vi "Tree_Get first enabled element from bottom.vi"(8 "error in (no error)":errorcluster, 11 "TreeControl Ref":refnum<vi>) -> (0 "error out":errorcluster, 2 "First Element Tag":string, 3 "Tree Control Ref Out":refnum<vi>)   [LabVIEW 2023]
doc: "Move from bottom of the tree up to find first non-dsiabled item in tree. This will open disabled parent items and traverse their children."
panel:
  in  "Tree":string[](tree)
  # "DEBUG CTRL"
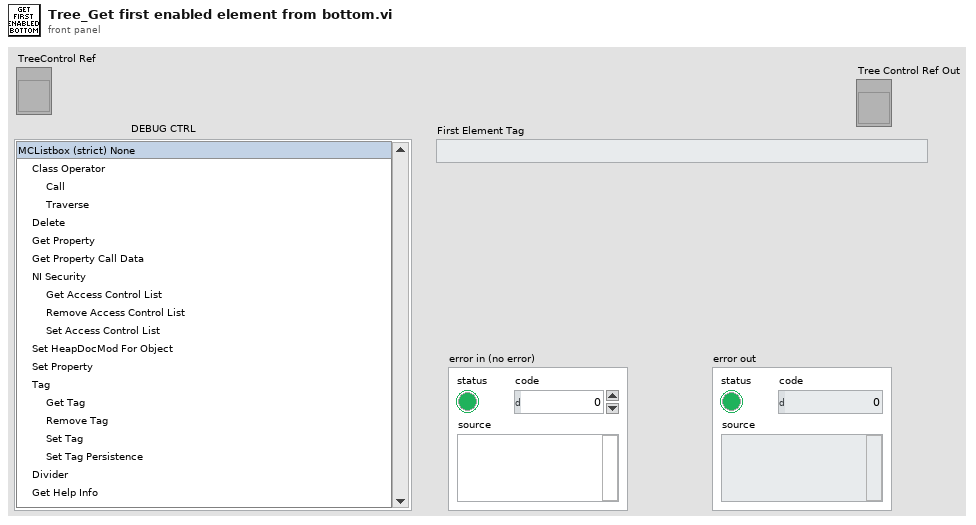
[diagram p1: front panel]
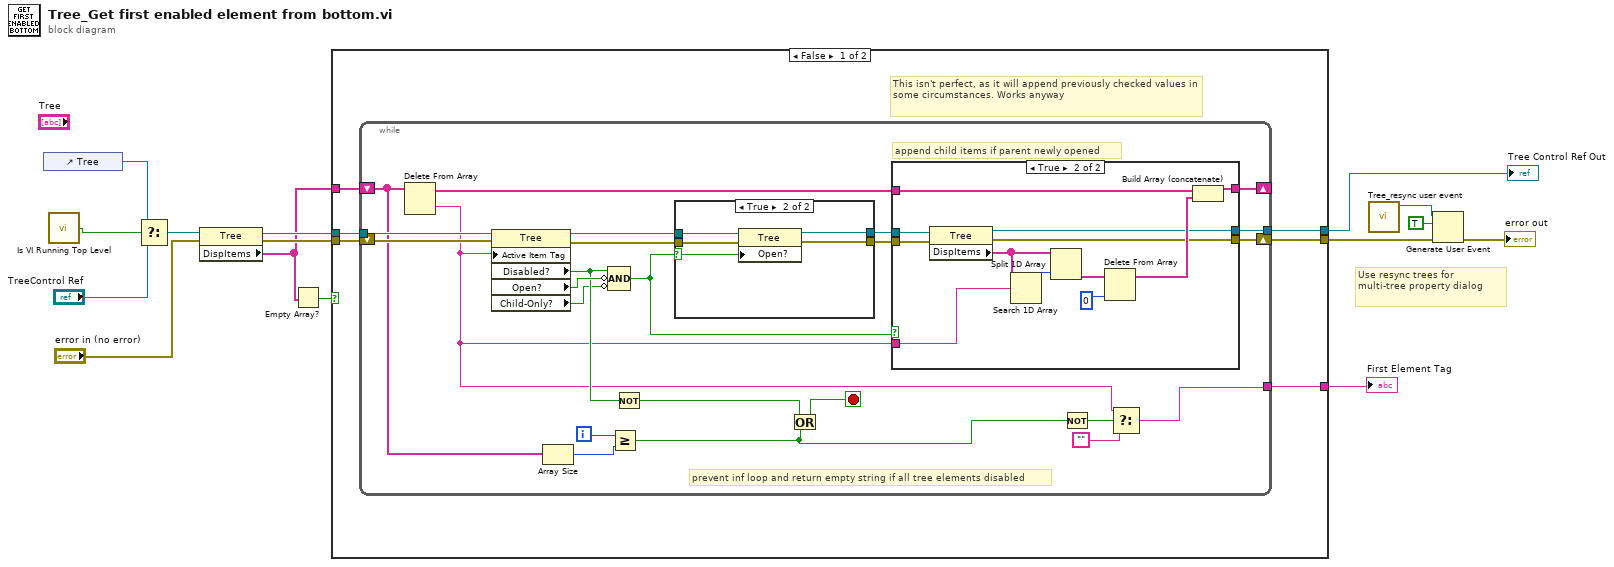
[diagram p0: block diagram]
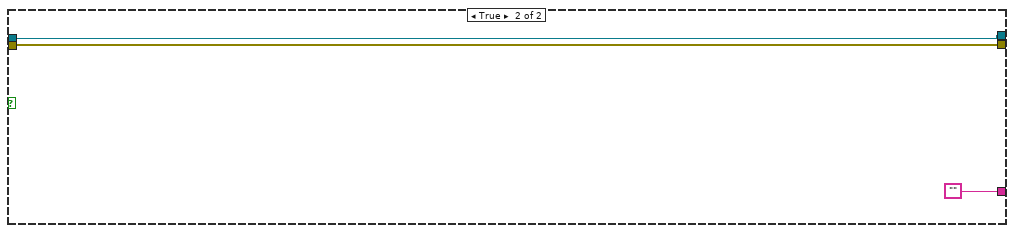
[diagram p4: hidden frame]
diagram:
  # "Use resync trees for multi-tree property dialog"
  n1 = control-ref of="Tree"() -> (w12:refnum<vi>)
  n2 = call "Is VI Running Top Level.vi"() -> ("Top Level?"=w13:bool)  [unwired: 5 in]
  n3 = Select(t=w12, s=w13, f="TreeControl Ref") -> (s? t:f=w10:refnum<vi>)
  n4 = property class="Tree"(reference=w10, error in="error in (no error)") -> (reference out=w15:refnum<vi>, error out=w9:errorcluster, "DispItems"=w2:string[])
  n5 = Empty Array?(array=w2) -> (empty?=w1:bool)
  n6 = case shown="False" w1 {
    tunnel: w15 -> [w21 w70]
    tunnel: w2 -> [w20 _]
    tunnel: [w19 ""] -> w14
    tunnel: w9 -> [w18 w69]
    tunnel: [w17 w70] -> w7
    tunnel: [w16 w69] -> w6
    frame False {
      # "This isn't perfect, as it will append previously checked values in some circumstances. Works anyway"
      n7 = while {
        tunnel: w21 -> [w43]
        tunnel: [w25] -> w19
        shift-right: [w39] -> _
        shift-left: w20 -> [w34]
        shift-right: [w35] -> w16
        shift-left: w18 -> [w38]
        tunnel: [w23] -> w17
        i -> [w33]
        stop <- w30 stop-if-true
        # "append child items if parent newly opened"
        # "prevent inf loop and return empty string if all tree elements disabled"
        n8 = Delete From Array(array=w34) -> (deleted portion=w26:string, array with subset deleted=w40:string[])  [unwired: 2 in]
        n9 = property class="Tree"(reference=w43, error in=w38, "Active Item Tag"=w26) -> (reference out=w45:refnum<vi>, error out=w37:errorcluster, "Disabled?"=w41:bool, "Open?"=w44:bool, "Child-Only?"=w24:bool)
        n10 = Array Size(array=w34) -> (size(s)=w32:i32)
        n11 = Compound Arithmetic op=AND(w41, invert w44, invert w24) -> (w22:bool)
        n12 = Greater Or Equal?(x=w33, y=w32) -> (x >= y?=w29:bool)
        n13 = Not(x=w41) -> (.not. x?=w31:bool)
        n14 = case shown="True" w22 {
          selector: w22 -> [_ w49]
          tunnel: w45 -> [w47 w52]
          tunnel: [w47 w51] -> w42
          tunnel: w37 -> [w46 w50]
          tunnel: [w46 w48] -> w36
          frame False {
          }
          frame True {
            n15 = property class="Tree"(reference=w52, error in=w50, "Open?"=w49) -> (reference out=w51:refnum<vi>, error out=w48:errorcluster)
          }
        }
        n16 = Or(x=w31, y=w29) -> (x .or. y?=w30:bool)
        n17 = case shown="True" w22 {
          tunnel: w42 -> [w53 w67]
          tunnel: w40 -> [w55 w61]
          tunnel: [w55 w60] -> w39
          tunnel: w36 -> [w54 w59]
          tunnel: [w54 w58] -> w35
          tunnel: w26 -> [_ w57]
          tunnel: [w53 w56] -> w23
          frame False {
          }
          frame True {
            n18 = property class="Tree"(reference=w67, error in=w59) -> (reference out=w56:refnum<vi>, error out=w58:errorcluster, "DispItems"=w66:string[])
            n19 = Search 1D Array(1D array=w66, element=w57) -> (index of element=w65:i32)  [unwired: 1 in]
            n20 = Split 1D Array(array=w66, index=w65) -> (second subarray=w64:string[])  [unwired: 1 out]
            n21 = Delete From Array(array=w64, index=0) -> (array with subset deleted=w62:string[])  [unwired: 1 in, 1 out]
            n22 = Build Array (concatenate)(w61, w62) -> (w60:string[])
          }
        }
        n23 = Not(x=w29) -> (.not. x?=w28:bool)
        n24 = Select(t=w26, s=w28, f="") -> (s? t:f=w25:string)
      }
    }
    frame True {
    }
  }
  "First Element Tag" <- w14
  "Tree Control Ref Out" <- w7
  n25 = call "Tree_resync user event.vi"() -> ("Open/close"=w4:refnum<user-event>)  [unwired: 11 in]
  n26 = Generate User Event(user event=w4, event data cluster=TRUE ("event data"), error in=w6) -> (error out=→"error out":errorcluster)  [unwired: 1 in, 1 out]
